vi "EnqueExperiments.vi"(0 "object in":refnum<class "ExperimentSeries2.lvclass">, 2 "element":refnum<class "Experiment2.lvclass">[](array[class]), 5 "error in (no error)":errorcluster) -> (14 "object out":refnum<class "ExperimentSeries2.lvclass">, 19 "error out":errorcluster)   [LabVIEW 2023, in "ExperimentSeries2.lvclass"]
uses:
  ExperimentSeries2.lvclass
  Experiment2_class/Experiment2.lvclass
  ExperimentSeries2.lvclass/ExperimentSeries2.ctl
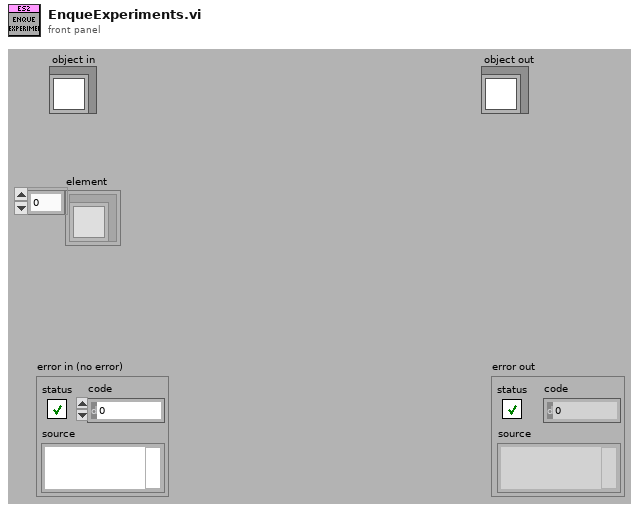
[diagram p1: front panel]
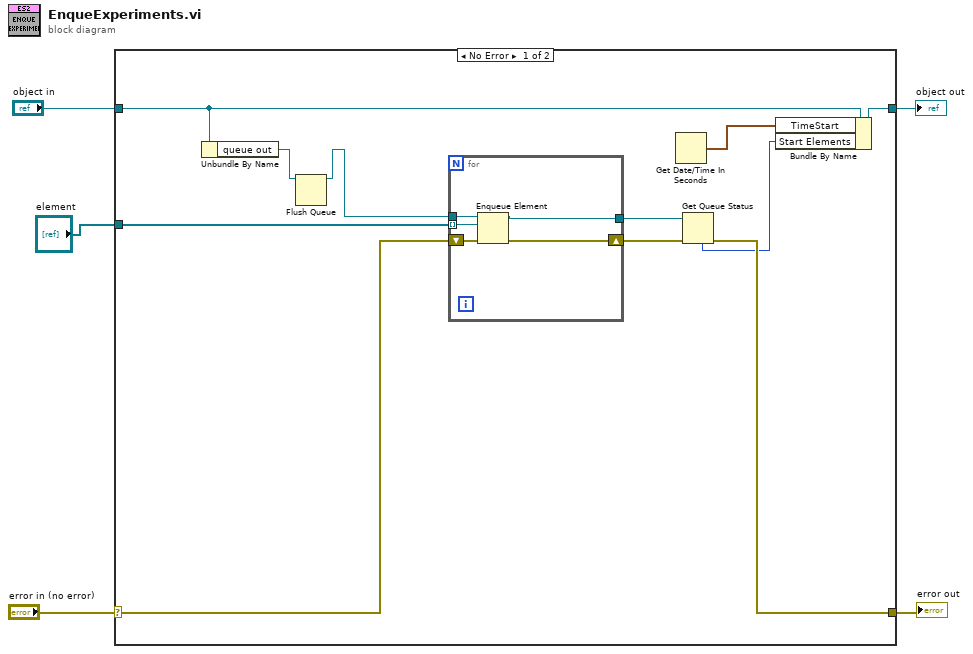
[diagram p0: block diagram]
diagram:
  n1 = case shown="No Error" "error in (no error)" {
    selector: "error in (no error)" -> [w14 w23]
    tunnel: [w10 w23] -> w4
    tunnel: [w8 w22] -> w2
    tunnel: "object in" -> [w16 w22]
    tunnel: "element" -> [w15 _]
    frame No Error {
      n2 = Unbundle By Name(w16) -> ("queue out"=w13:refnum<queue>)
      n3 = Flush Queue(queue=w13) -> (queue out=w12:refnum<queue>)  [unwired: 1 in, 2 out]
      n4 = for {
        tunnel: w12 -> [w21]
        tunnel: w15 -> [w19] mode=indexing
        shift-right: [w18] -> w11
        shift-left: w14 -> [w20]
        tunnel: [w17] -> w9
        n5 = Enqueue Element(queue=w21, element=w19, error in (no error)=w20) -> (queue out=w17:refnum<queue>, error out=w18:errorcluster)  [unwired: 1 in, 1 out]
      }
      n6 = Get Date/Time In Seconds() -> (seconds since 1Jan1904=w7:timestamp)
      n7 = Get Queue Status(queue=w9, error in (no error)=w11) -> (error out=w10:errorcluster, # elements in queue=w6:i32)  [unwired: 1 in, 6 out]
      n8 = Bundle By Name(cluster=w16, "TimeStart"=w7, "Start Elements"=w6) -> (w8:refnum<class "ExperimentSeries2.lvclass">)
    }
    frame Error {
    }
  }
  "error out" <- w4
  "object out" <- w2
